vi "RoomsFGV.vi"(7 "Actions":T1, 8 "error in (no error)":errorcluster, 9 "Data In":string, 10 "Room":i32) -> (0 "error out":errorcluster, 1 "Data Out":string)   [LabVIEW 2015]
uses:
  TypeDef/RoomsActionEnum.ctl
  TypeDef/RoomsStateCluster.ctl
  LVClasses/Room/Room.lvclass
  LVClasses/Room/Room.lvclass/Room.ctl
  LVClasses/Flags/Flags.lvclass/Flags.ctl
  LVClasses/Request/SummaryJsonCluster.ctl
  LVClasses/Room/Write Bed URL.vi
  LVClasses/Room/Read Flags.lvclass.vi
  LVClasses/Room/Read RoomRequests.vi
  LVClasses/Room/Read InRoomPersonnel.vi
  LVClasses/Room/Read Beacon Id.vi
  LVClasses/Room/Read Bed URL.vi
  LVClasses/Room/Read Room Number.vi
  LVClasses/Room/Read BedVacant.vi
  LVClasses/Flags/Read State.vi
  LVClasses/Flags/Write State.vi
  LVClasses/Room/Write Flags.lvclass.vi
  LVClasses/Room/Write BedVacant.vi
  LVClasses/Room/Write RoomRequests.vi
  LVClasses/Room/Write InRoomPersonnel.vi
  <vilib>/Utility/error.llb/Error Cluster From Error Code.vi
  <vilib>/ErrorRing/Error Ring.xnode
  LVClasses/Flags/Flags.lvclass
  LVClasses/Request/Request.lvclass
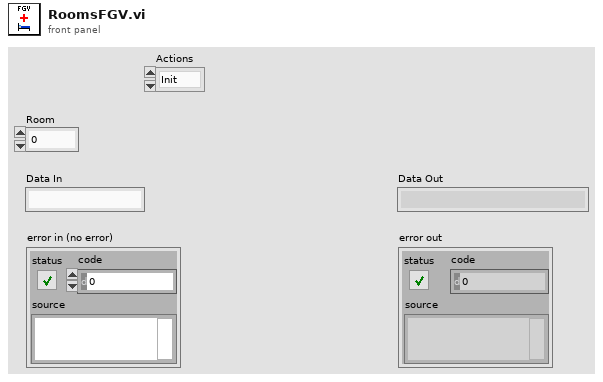
[diagram p1: front panel]
types:
  T1 = typedef "RoomsActionEnum.ctl" = enum16{"Init", "Add Room", "Remove Room", "Read Room", "Read Flag", "Read Flag State", "Write Flag State", "Read Flag Color", "Write Flag Color", "Read Bed Vacant", "Write Bed Vacant", "Read Personnel", "Add Personnel", "Remove Personnel", "Read Requests", "Add Request", "Remove Request", "Read Beacon ID", "Write Beacon ID", "Write Bed URL", "Read Bed URL", "Read Rooms Numbers", "Write Flag"}
  T2 = typedef "RoomsStateCluster.ctl" = cluster{"Rooms":refnum<class "Room.lvclass">[]}
  T3 = typedef "Request.lvclass/SummaryJsonCluster.ctl" = cluster{"RequestID":string, "EnlapsedTime":i32, "Description":string, "Alarm":bool}
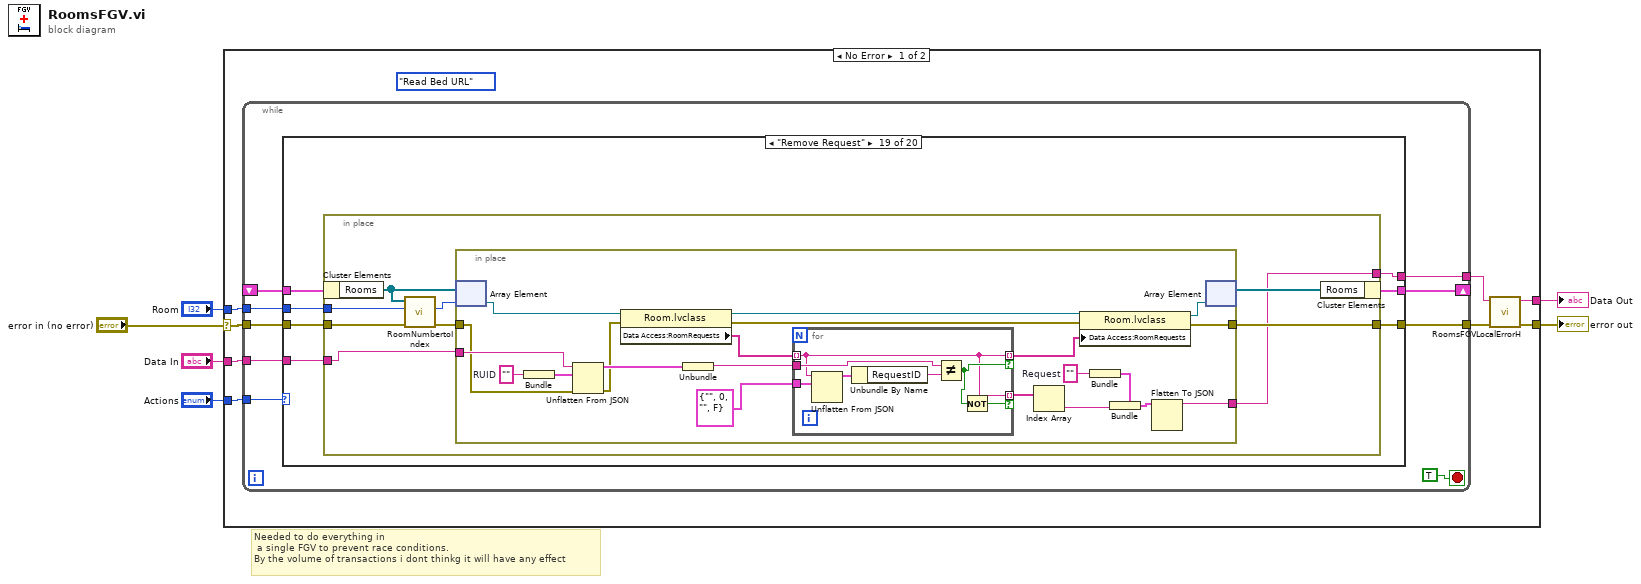
[diagram p0: block diagram]
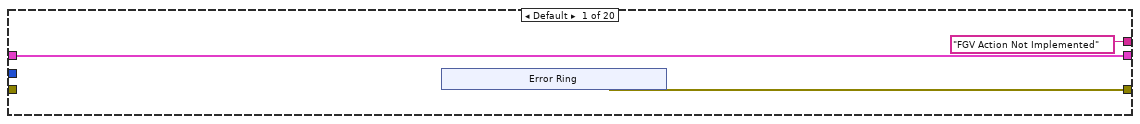
[diagram p2: hidden frame]
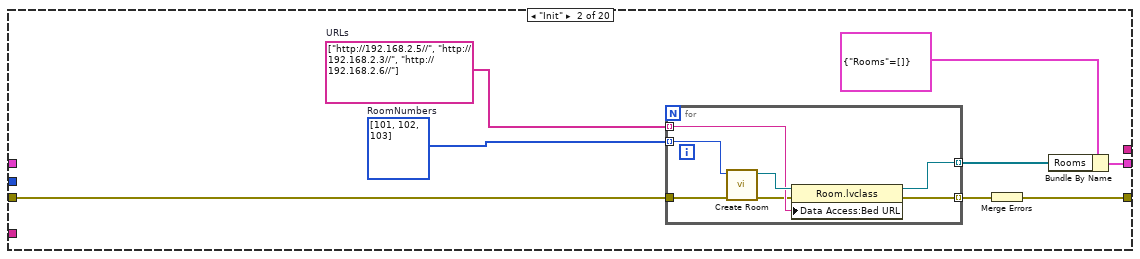
[diagram p3: hidden frame]
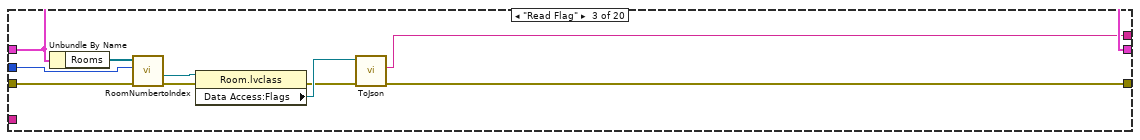
[diagram p4: hidden frame]
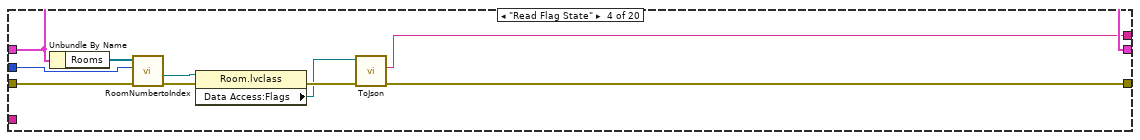
[diagram p5: hidden frame]
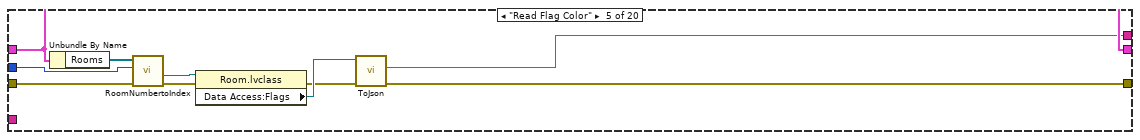
[diagram p6: hidden frame]
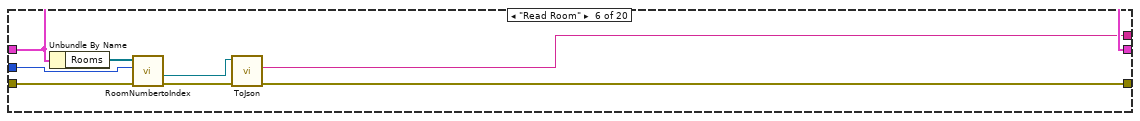
[diagram p7: hidden frame]
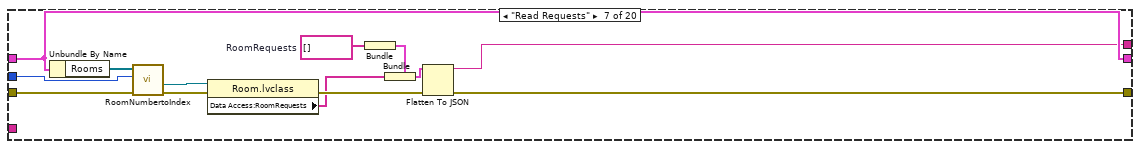
[diagram p8: hidden frame]
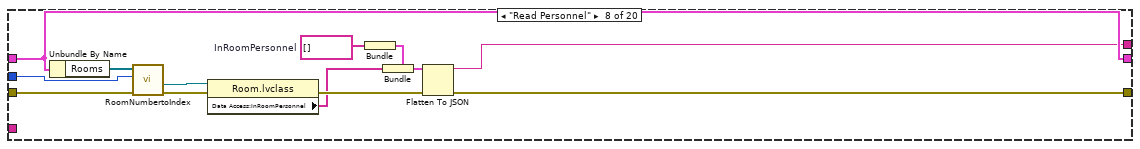
[diagram p9: hidden frame]
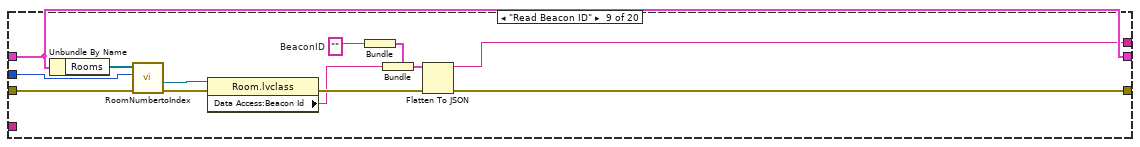
[diagram p10: hidden frame]
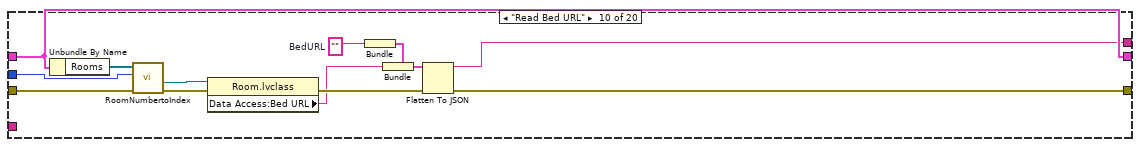
[diagram p11: hidden frame]
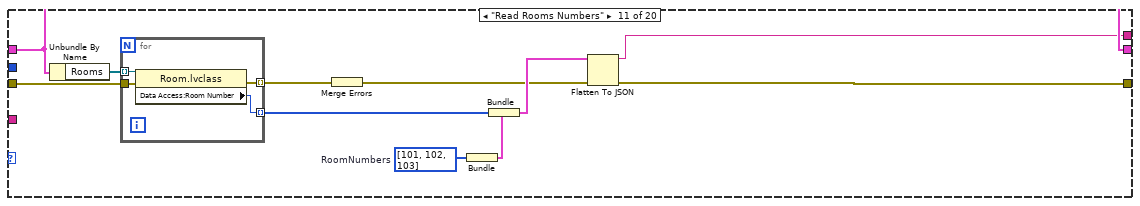
[diagram p12: hidden frame]
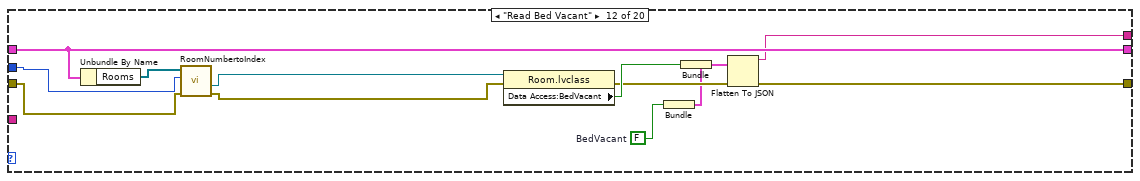
[diagram p13: hidden frame]
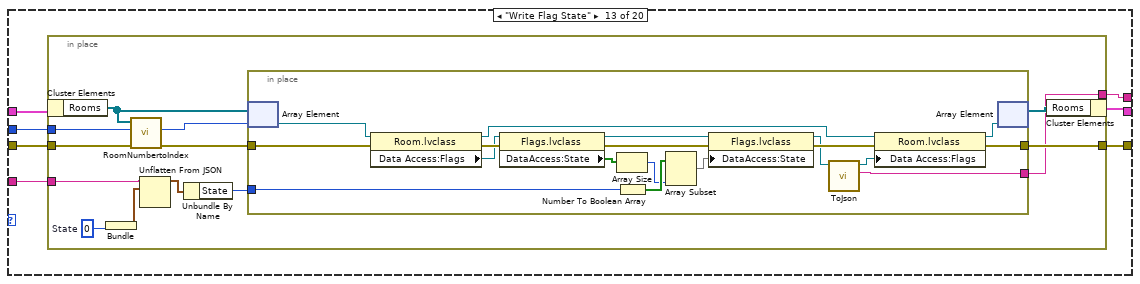
[diagram p14: hidden frame]
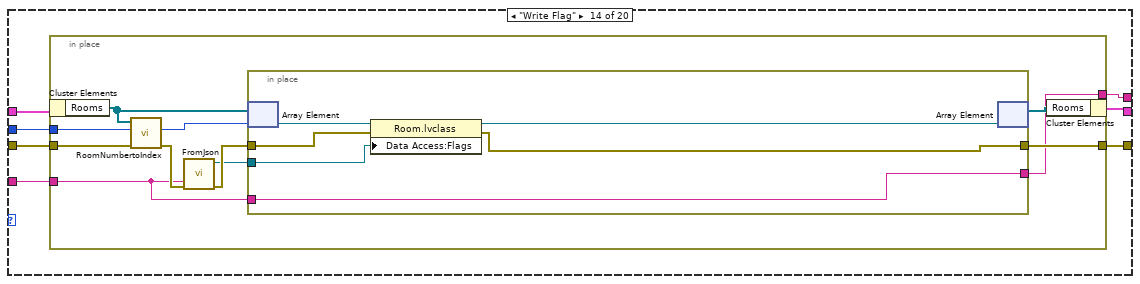
[diagram p15: hidden frame]
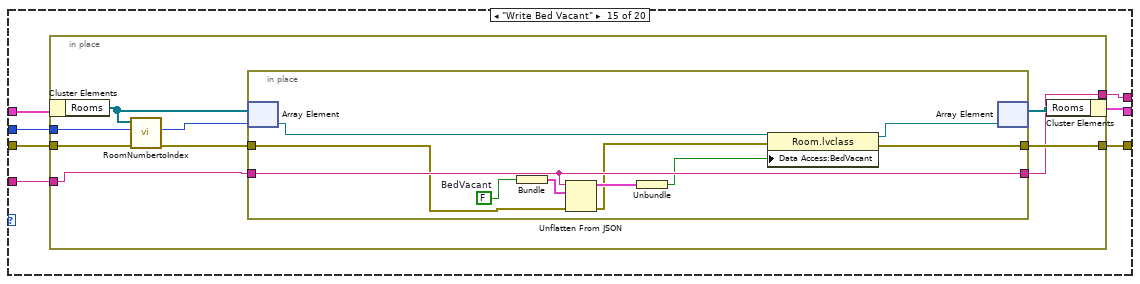
[diagram p16: hidden frame]
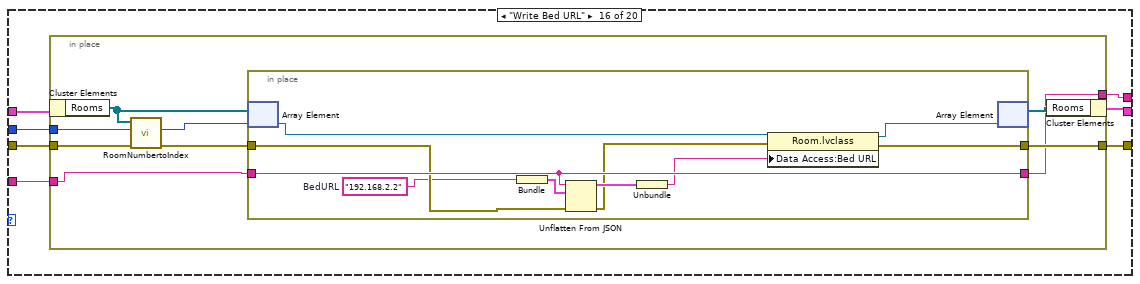
[diagram p17: hidden frame]
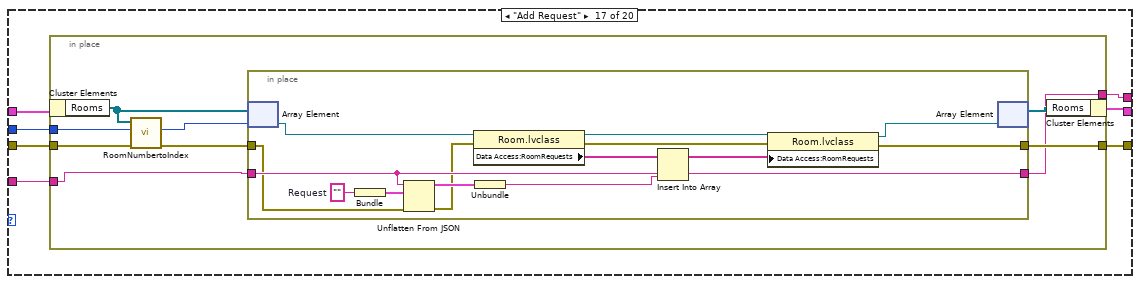
[diagram p18: hidden frame]
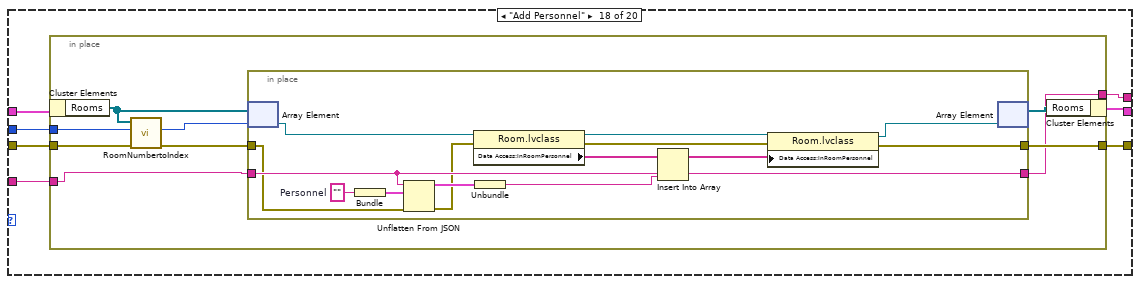
[diagram p19: hidden frame]
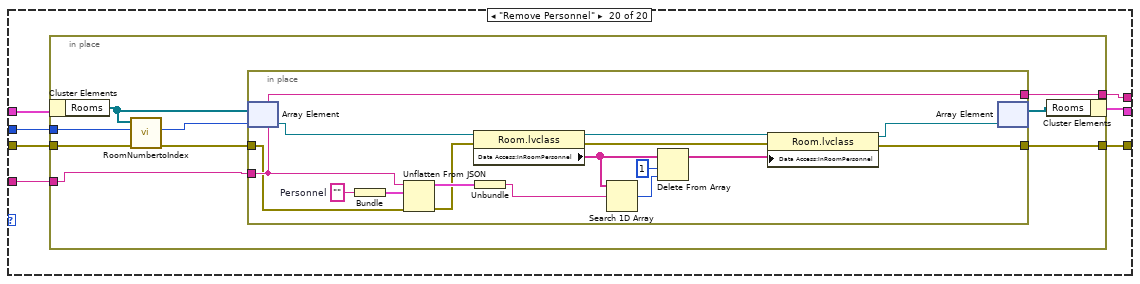
[diagram p20: hidden frame]
diagram:
  # "Needed to do everything in\n a single FGV to prevent race conditions. \nBy the volume of transactions i dont thinkg it will have any effect"
  n1 = case shown="No Error" "error in (no error)" {
    selector: "error in (no error)" -> [w11 w415]
    tunnel: "Actions" -> [w14 _]
    tunnel: "Room" -> [w13 _]
    tunnel: [w9 _] -> w4
    tunnel: "Data In" -> [w12 _]
    tunnel: [w10 w415] -> w1
    frame No Error {
      (unwired) RoomsActionEnum."Read Bed URL" ("Actions")
      n2 = while {
        shift-right: [w21] -> _
        shift-left: _ -> [w20]
        tunnel: w14 -> [w22]
        tunnel: w13 -> [w19]
        tunnel: [w18] -> w8
        tunnel: w12 -> [w17]
        tunnel: [w16] -> w7
        tunnel: w11 -> [w15]
        stop <- TRUE ("stop") stop-if-true
        n3 = case shown="\"Remove Request\"" w22 {
          tunnel: [w26 w39 w56 w66 w76 w84 w97 w110 w123 w136 w147 w164 w170 w208 w232 w258 w284 w314 w344 w388] -> w21
          tunnel: w20 -> [w26 _ w56 w66 w76 w84 w97 w110 w123 w136 w147 w164 w171 w209 w233 w259 w285 w315 w345 w389]
          tunnel: w19 -> [_ _ w55 w65 w75 w83 w96 w109 w122 w135 _ w155 w169 w207 w231 w257 w283 w313 w343 w387]
          tunnel: ["FGV Action Not Implemented" ("Data In") _ w51 w61 w71 w78 w91 w104 w117 w130 w145 w162 w168 w206 w230 w256 w282 w312 w342 w386] -> w18
          tunnel: w17 -> [_ _ _ _ _ _ _ _ _ _ _ _ w166 w204 w228 w254 w280 w310 w340 w384]
          tunnel: [w24 w32 w47 w57 w67 w77 w85 w98 w112 w125 w137 w157 w165 w203 w227 w253 w279 w309 w339 w383] -> w16
          tunnel: w15 -> [_ w33 w52 w62 w72 w81 w94 w107 w120 w133 w140 w154 w167 w205 w229 w255 w281 w311 w341 w385]
          frame Default {
            n4 = xnode "Error Ring"() -> ("error out"=w24:errorcluster)
          }
          frame "Init" {
            w36 = i32[] [101, 102, 103]  # RoomNumbers
            w35 = string[] ["http://192.168.2.5//", "http://192.168.2.3//", "http://192.168.2.6//"]  # URLs
            n5 = for {
              tunnel: w36 -> [w40] mode=indexing
              tunnel: [w45] -> w37 mode=indexing
              tunnel: w35 -> [w44] mode=indexing
              tunnel: w33 -> [w42]
              tunnel: [w41] -> w34 mode=indexing
              n6 = call "Create Room.vi"("error in"=w42, "Room Number"=w40) -> ("error out"=w43:errorcluster, "Room Ref"=w46:refnum<class "Room.lvclass">)  [unwired: 8 in]
              n7 = property class="Room.lvclass"(reference=w46, error in=w43, "Data Access:Bed URL"=w44) -> (reference out=w45:refnum<class "Room.lvclass">, error out=w41:errorcluster)
            }
            n8 = Merge Errors(w34) -> (w32:errorcluster)
            n9 = Bundle By Name(cluster=T2 {"Rooms"=[]}, "Rooms"=w37) -> (w39:T2)
          }
          frame "Read Flag" {
            n10 = Unbundle By Name(w56) -> ("Rooms"=w54:refnum<class "Room.lvclass">[])
            n11 = call "RoomNumbertoIndex.vi"("error in (no error)"=w52, "y"=w55, "Rooms In"=w54) -> ("error out"=w48:errorcluster, "Room"=w53:refnum<class "Room.lvclass">)  [unwired: 5 in, 2 out]
            n12 = property class="Room.lvclass"(reference=w53, error in=w48) -> (error out=w49:errorcluster, "Data Access:Flags"=w50:refnum<class "Flags.lvclass">)  [unwired: 1 out]
            n13 = call "ToJson.vi"("error in (no error)"=w49, "Flags in"=w50) -> ("error out"=w47:errorcluster, "String"=w51:string)  [unwired: 7 in, 1 out]
          }
          frame "Read Flag State" {
            n14 = Unbundle By Name(w66) -> ("Rooms"=w64:refnum<class "Room.lvclass">[])
            n15 = call "RoomNumbertoIndex.vi"("error in (no error)"=w62, "y"=w65, "Rooms In"=w64) -> ("error out"=w59:errorcluster, "Room"=w63:refnum<class "Room.lvclass">)  [unwired: 5 in, 2 out]
            n16 = property class="Room.lvclass"(reference=w63, error in=w59) -> (error out=w60:errorcluster, "Data Access:Flags"=w58:refnum<class "Flags.lvclass">)  [unwired: 1 out]
            n17 = call "ToJson.vi"("error in (no error)"=w60, "Flags in"=w58) -> ("error out"=w57:errorcluster, "String"=w61:string)  [unwired: 7 in, 1 out]
          }
          frame "Read Flag Color" {
            n18 = Unbundle By Name(w76) -> ("Rooms"=w74:refnum<class "Room.lvclass">[])
            n19 = call "RoomNumbertoIndex.vi"("error in (no error)"=w72, "y"=w75, "Rooms In"=w74) -> ("error out"=w68:errorcluster, "Room"=w73:refnum<class "Room.lvclass">)  [unwired: 5 in, 2 out]
            n20 = property class="Room.lvclass"(reference=w73, error in=w68) -> (error out=w69:errorcluster, "Data Access:Flags"=w70:refnum<class "Flags.lvclass">)  [unwired: 1 out]
            n21 = call "ToJson.vi"("error in (no error)"=w69, "Flags in"=w70) -> ("error out"=w67:errorcluster, "String"=w71:string)  [unwired: 7 in, 1 out]
          }
          frame "Read Room" {
            n22 = Unbundle By Name(w84) -> ("Rooms"=w82:refnum<class "Room.lvclass">[])
            n23 = call "RoomNumbertoIndex.vi"("error in (no error)"=w81, "y"=w83, "Rooms In"=w82) -> ("error out"=w80:errorcluster, "Room"=w79:refnum<class "Room.lvclass">)  [unwired: 5 in, 2 out]
            n24 = call "ToJson.vi"("error in (no error)"=w80, "Room in"=w79) -> ("error out"=w77:errorcluster, "String"=w78:string)  [unwired: 7 in, 1 out]
          }
          frame "Read Requests" {
            w88 = string[] []  # RoomRequests
            n25 = Unbundle By Name(w97) -> ("Rooms"=w95:refnum<class "Room.lvclass">[])
            n26 = call "RoomNumbertoIndex.vi"("error in (no error)"=w94, "y"=w96, "Rooms In"=w95) -> ("error out"=w92:errorcluster, "Room"=w93:refnum<class "Room.lvclass">)  [unwired: 5 in, 2 out]
            n27 = property class="Room.lvclass"(reference=w93, error in=w92) -> (error out=w90:errorcluster, "Data Access:RoomRequests"=w86:string[])  [unwired: 1 out]
            n28 = Bundle("RoomRequests"=w88) -> (w89:cluster{"RoomRequests":string[]})  [unwired: 1 in]
            n29 = Bundle(cluster=w89, "RoomRequests"=w86) -> (w87:cluster{"RoomRequests":string[]})
            n30 = Flatten To JSON(anything=w87, error in (no error)=w90) -> (JSON string=w91:string, 11:w85:errorcluster)  [unwired: 1 in]
          }
          frame "Read Personnel" {
            w101 = string[] []  # InRoomPersonnel
            n31 = Unbundle By Name(w110) -> ("Rooms"=w108:refnum<class "Room.lvclass">[])
            n32 = call "RoomNumbertoIndex.vi"("error in (no error)"=w107, "y"=w109, "Rooms In"=w108) -> ("error out"=w105:errorcluster, "Room"=w106:refnum<class "Room.lvclass">)  [unwired: 5 in, 2 out]
            n33 = property class="Room.lvclass"(reference=w106, error in=w105) -> (error out=w103:errorcluster, "Data Access:InRoomPersonnel"=w99:string[])  [unwired: 1 out]
            n34 = Bundle("InRoomPersonnel"=w101) -> (w102:cluster{"InRoomPersonnel":string[]})  [unwired: 1 in]
            n35 = Bundle(cluster=w102, "InRoomPersonnel"=w99) -> (w100:cluster{"InRoomPersonnel":string[]})
            n36 = Flatten To JSON(anything=w100, error in (no error)=w103) -> (JSON string=w104:string, 11:w98:errorcluster)  [unwired: 1 in]
          }
          frame "Read Beacon ID" {
            w111 = ""  # BeaconID
            n37 = Unbundle By Name(w123) -> ("Rooms"=w121:refnum<class "Room.lvclass">[])
            n38 = call "RoomNumbertoIndex.vi"("error in (no error)"=w120, "y"=w122, "Rooms In"=w121) -> ("error out"=w118:errorcluster, "Room"=w119:refnum<class "Room.lvclass">)  [unwired: 5 in, 2 out]
            n39 = property class="Room.lvclass"(reference=w119, error in=w118) -> (error out=w116:errorcluster, "Data Access:Beacon Id"=w113:string)  [unwired: 1 out]
            n40 = Bundle("BeaconID"=w111) -> (w115:cluster{"BeaconID":string})  [unwired: 1 in]
            n41 = Bundle(cluster=w115, "BeaconID"=w113) -> (w114:cluster{"BeaconID":string})
            n42 = Flatten To JSON(anything=w114, error in (no error)=w116) -> (JSON string=w117:string, 11:w112:errorcluster)  [unwired: 1 in]
          }
          frame "Read Bed URL" {
            w124 = ""  # BedURL
            n43 = Unbundle By Name(w136) -> ("Rooms"=w134:refnum<class "Room.lvclass">[])
            n44 = call "RoomNumbertoIndex.vi"("error in (no error)"=w133, "y"=w135, "Rooms In"=w134) -> ("error out"=w131:errorcluster, "Room"=w132:refnum<class "Room.lvclass">)  [unwired: 5 in, 2 out]
            n45 = property class="Room.lvclass"(reference=w132, error in=w131) -> (error out=w129:errorcluster, "Data Access:Bed URL"=w126:string)  [unwired: 1 out]
            n46 = Bundle("BedURL"=w124) -> (w128:cluster{"BedURL":string})  [unwired: 1 in]
            n47 = Bundle(cluster=w128, "BedURL"=w126) -> (w127:cluster{"BedURL":string})
            n48 = Flatten To JSON(anything=w127, error in (no error)=w129) -> (JSON string=w130:string, 11:w125:errorcluster)  [unwired: 1 in]
          }
          frame "Read Rooms Numbers" {
            w146 = i32[] [101, 102, 103]  # RoomNumbers
            n49 = Unbundle By Name(w147) -> ("Rooms"=w142:refnum<class "Room.lvclass">[])
            n50 = for {
              tunnel: w142 -> [w151] mode=indexing
              tunnel: [w150] -> w141 mode=indexing
              tunnel: w140 -> [w149]
              tunnel: [w148] -> w139 mode=indexing
              n51 = property class="Room.lvclass"(reference=w151, error in=w149) -> (error out=w148:errorcluster, "Data Access:Room Number"=w150:i32)  [unwired: 1 out]
            }
            n52 = Merge Errors(w139) -> (w138:errorcluster)
            n53 = Bundle("RoomNumbers"=w146) -> (w144:cluster{"RoomNumbers":i32[]})  [unwired: 1 in]
            n54 = Bundle(cluster=w144, "RoomNumbers"=w141) -> (w143:cluster{"RoomNumbers":i32[]})
            n55 = Flatten To JSON(anything=w143, error in (no error)=w138) -> (JSON string=w145:string, 11:w137:errorcluster)  [unwired: 1 in]
          }
          frame "Read Bed Vacant" {
            w159 = FALSE  # BedVacant
            n56 = Unbundle By Name(w164) -> ("Rooms"=w156:refnum<class "Room.lvclass">[])
            n57 = call "RoomNumbertoIndex.vi"("error in (no error)"=w154, "y"=w155, "Rooms In"=w156) -> ("error out"=w153:errorcluster, "Room"=w152:refnum<class "Room.lvclass">)  [unwired: 5 in, 2 out]
            n58 = property class="Room.lvclass"(reference=w152, error in=w153) -> (error out=w160:errorcluster, "Data Access:BedVacant"=w161:bool)  [unwired: 1 out]
            n59 = Bundle("BedVacant"=w159) -> (w158:cluster{"BedVacant":bool})  [unwired: 1 in]
            n60 = Bundle(cluster=w158, "BedVacant"=w161) -> (w163:cluster{"BedVacant":bool})
            n61 = Flatten To JSON(anything=w163, error in (no error)=w160) -> (JSON string=w162:string, 11:w157:errorcluster)  [unwired: 1 in]
          }
          frame "Write Flag State" {
            n62 = in-place {
              in-place-border: w169 -> [w182]
              in-place-border: [w178] -> w168
              in-place-border: w167 -> [w180]
              in-place-border: [w179] -> w165
              in-place-border: w166 -> [w176]
              w175 = 0  # State
              n63 = in-place-cluster #1(w171) -> ("Rooms"=w183:refnum<class "Room.lvclass">[])
              n64 = Bundle("State"=w175) -> (w174:cluster{"State":i32})  [unwired: 1 in]
              n65 = call "RoomNumbertoIndex.vi"("error in (no error)"=w180, "y"=w182, "Rooms In"=w183) -> ("error out"=w177:errorcluster, "Index"=w181:i32)  [unwired: 5 in, 2 out]
              n66 = Unflatten From JSON(JSON string=w176, type and defaults=w174) -> (value=w173:cluster{"State":i32})  [unwired: 5 in, 1 out]
              n67 = Unbundle By Name(w173) -> ("State"=w172:i32)
              n68 = in-place {
                in-place-border: w177 -> [w197]
                in-place-border: [w189] -> w179
                in-place-border: w172 -> [w200]
                in-place-border: [w185] -> w178
                n69 = in-place-array #2(w183, w181) -> (w192:refnum<class "Room.lvclass">)
                n70 = property class="Room.lvclass"(reference=w192, error in=w197) -> (reference out=w191:refnum<class "Room.lvclass">, error out=w198:errorcluster, "Data Access:Flags"=w196:refnum<class "Flags.lvclass">)
                n71 = property class="Flags.lvclass"(reference=w196, error in=w198) -> (reference out=w188:refnum<class "Flags.lvclass">, error out=w199:errorcluster, "DataAccess:State"=w195:bool[])
                n72 = Array Size(array=w195) -> (size(s)=w194:i32)
                n73 = Number To Boolean Array(number=w200) -> (Boolean array=w201:bool[])
                n74 = Array Subset(array=w201, length=w194) -> (w193:bool[])  [unwired: 1 in]
                n75 = property class="Flags.lvclass"(reference=w188, error in=w199, "DataAccess:State"=w193) -> (reference out=w187:refnum<class "Flags.lvclass">, error out=w190:errorcluster)
                n76 = call "ToJson.vi"("Flags in"=w187) -> ("String"=w185:string, "Flags out"=w186:refnum<class "Flags.lvclass">)  [unwired: 8 in, 1 out]
                n77 = property class="Room.lvclass"(reference=w191, error in=w190, "Data Access:Flags"=w186) -> (reference out=w202:refnum<class "Room.lvclass">, error out=w189:errorcluster)
                n78 = in-place-array #2(w202) -> (w184:refnum<class "Room.lvclass">[])  [unwired: 1 out]
              }
              n79 = in-place-cluster #1("Rooms"=w184) -> (w170:T2)
            }
          }
          frame "Write Flag" {
            n80 = in-place {
              in-place-border: w207 -> [w218]
              in-place-border: [w214] -> w206
              in-place-border: w205 -> [w216]
              in-place-border: [w215] -> w203
              in-place-border: w204 -> [w211]
              n81 = in-place-cluster #3(w209) -> ("Rooms"=w219:refnum<class "Room.lvclass">[])
              n82 = call "RoomNumbertoIndex.vi"("error in (no error)"=w216, "y"=w218, "Rooms In"=w219) -> ("error out"=w213:errorcluster, "Index"=w217:i32)  [unwired: 5 in, 2 out]
              n83 = call "FromJson.vi"("error in (no error)"=w213, "String"=w211) -> ("error out"=w212:errorcluster, "Flags out"=w210:refnum<class "Flags.lvclass">)  [unwired: 8 in]
              n84 = in-place {
                in-place-border: w212 -> [w226]
                in-place-border: [w223] -> w215
                in-place-border: [w224] -> w214
                in-place-border: w211 -> [w224]
                in-place-border: w210 -> [w221]
                n85 = in-place-array #4(w219, w217) -> (w225:refnum<class "Room.lvclass">)
                n86 = property class="Room.lvclass"(reference=w225, error in=w226, "Data Access:Flags"=w221) -> (reference out=w222:refnum<class "Room.lvclass">, error out=w223:errorcluster)
                n87 = in-place-array #4(w222) -> (w220:refnum<class "Room.lvclass">[])  [unwired: 1 out]
              }
              n88 = in-place-cluster #3("Rooms"=w220) -> (w208:T2)
            }
          }
          frame "Write Bed Vacant" {
            n89 = in-place {
              in-place-border: w231 -> [w240]
              in-place-border: [w236] -> w230
              in-place-border: w229 -> [w238]
              in-place-border: [w237] -> w227
              in-place-border: w228 -> [w235]
              n90 = in-place-cluster #5(w233) -> ("Rooms"=w241:refnum<class "Room.lvclass">[])
              n91 = call "RoomNumbertoIndex.vi"("error in (no error)"=w238, "y"=w240, "Rooms In"=w241) -> ("error out"=w234:errorcluster, "Index"=w239:i32)  [unwired: 5 in, 2 out]
              n92 = in-place {
                in-place-border: w234 -> [w243]
                in-place-border: [w252] -> w237
                in-place-border: [w249] -> w236
                in-place-border: w235 -> [w249]
                w246 = FALSE  # BedVacant
                n93 = in-place-array #6(w241, w239) -> (w245:refnum<class "Room.lvclass">)
                n94 = Bundle("BedVacant"=w246) -> (w250:cluster{"BedVacant":bool})  [unwired: 1 in]
                n95 = Unflatten From JSON(JSON string=w249, type and defaults=w250, error in (no error)=w243) -> (value=w248:cluster{"BedVacant":bool}, error out=w244:errorcluster)  [unwired: 4 in]
                n96 = Unbundle(w248) -> ("BedVacant"=w247:bool)
                n97 = property class="Room.lvclass"(reference=w245, error in=w244, "Data Access:BedVacant"=w247) -> (reference out=w251:refnum<class "Room.lvclass">, error out=w252:errorcluster)
                n98 = in-place-array #6(w251) -> (w242:refnum<class "Room.lvclass">[])  [unwired: 1 out]
              }
              n99 = in-place-cluster #5("Rooms"=w242) -> (w232:T2)
            }
          }
          frame "Write Bed URL" {
            n100 = in-place {
              in-place-border: w257 -> [w266]
              in-place-border: [w262] -> w256
              in-place-border: w255 -> [w264]
              in-place-border: [w263] -> w253
              in-place-border: w254 -> [w261]
              n101 = in-place-cluster #7(w259) -> ("Rooms"=w267:refnum<class "Room.lvclass">[])
              n102 = call "RoomNumbertoIndex.vi"("error in (no error)"=w264, "y"=w266, "Rooms In"=w267) -> ("error out"=w260:errorcluster, "Index"=w265:i32)  [unwired: 5 in, 2 out]
              n103 = in-place {
                in-place-border: w260 -> [w270]
                in-place-border: [w278] -> w263
                in-place-border: [w275] -> w262
                in-place-border: w261 -> [w275]
                w269 = "192.168.2.2"  # BedURL
                n104 = in-place-array #8(w267, w265) -> (w272:refnum<class "Room.lvclass">)
                n105 = Bundle("BedURL"=w269) -> (w276:cluster{"BedURL":string})  [unwired: 1 in]
                n106 = Unflatten From JSON(JSON string=w275, type and defaults=w276, error in (no error)=w270) -> (value=w274:cluster{"BedURL":string}, error out=w271:errorcluster)  [unwired: 4 in]
                n107 = Unbundle(w274) -> ("BedURL"=w273:string)
                n108 = property class="Room.lvclass"(reference=w272, error in=w271, "Data Access:Bed URL"=w273) -> (reference out=w277:refnum<class "Room.lvclass">, error out=w278:errorcluster)
                n109 = in-place-array #8(w277) -> (w268:refnum<class "Room.lvclass">[])  [unwired: 1 out]
              }
              n110 = in-place-cluster #7("Rooms"=w268) -> (w258:T2)
            }
          }
          frame "Add Request" {
            n111 = in-place {
              in-place-border: w283 -> [w292]
              in-place-border: [w288] -> w282
              in-place-border: w281 -> [w290]
              in-place-border: [w289] -> w279
              in-place-border: w280 -> [w287]
              n112 = in-place-cluster #9(w285) -> ("Rooms"=w293:refnum<class "Room.lvclass">[])
              n113 = call "RoomNumbertoIndex.vi"("error in (no error)"=w290, "y"=w292, "Rooms In"=w293) -> ("error out"=w286:errorcluster, "Index"=w291:i32)  [unwired: 5 in, 2 out]
              n114 = in-place {
                in-place-border: w286 -> [w302]
                in-place-border: [w308] -> w289
                in-place-border: [w305] -> w288
                in-place-border: w287 -> [w305]
                w301 = ""  # Request
                n115 = in-place-array #10(w293, w291) -> (w303:refnum<class "Room.lvclass">)
                n116 = Bundle("Request"=w301) -> (w306:cluster{"Request":string})  [unwired: 1 in]
                n117 = Unflatten From JSON(JSON string=w305, type and defaults=w306, error in (no error)=w302) -> (value=w304:cluster{"Request":string}, error out=w299:errorcluster)  [unwired: 4 in]
                n118 = property class="Room.lvclass"(reference=w303, error in=w299) -> (reference out=w300:refnum<class "Room.lvclass">, error out=w298:errorcluster, "Data Access:RoomRequests"=w297:string[])
                n119 = Unbundle(w304) -> ("Request"=w295:string)
                n120 = Insert Into Array(array=w297, new element=w295) -> (w296:string[])  [unwired: 1 in]
                n121 = property class="Room.lvclass"(reference=w300, error in=w298, "Data Access:RoomRequests"=w296) -> (reference out=w307:refnum<class "Room.lvclass">, error out=w308:errorcluster)
                n122 = in-place-array #10(w307) -> (w294:refnum<class "Room.lvclass">[])  [unwired: 1 out]
              }
              n123 = in-place-cluster #9("Rooms"=w294) -> (w284:T2)
            }
          }
          frame "Add Personnel" {
            n124 = in-place {
              in-place-border: w313 -> [w322]
              in-place-border: [w318] -> w312
              in-place-border: w311 -> [w320]
              in-place-border: [w319] -> w309
              in-place-border: w310 -> [w317]
              n125 = in-place-cluster #11(w315) -> ("Rooms"=w323:refnum<class "Room.lvclass">[])
              n126 = call "RoomNumbertoIndex.vi"("error in (no error)"=w320, "y"=w322, "Rooms In"=w323) -> ("error out"=w316:errorcluster, "Index"=w321:i32)  [unwired: 5 in, 2 out]
              n127 = in-place {
                in-place-border: w316 -> [w332]
                in-place-border: [w338] -> w319
                in-place-border: [w335] -> w318
                in-place-border: w317 -> [w335]
                w331 = ""  # Personnel
                n128 = in-place-array #12(w323, w321) -> (w333:refnum<class "Room.lvclass">)
                n129 = Bundle("Personnel"=w331) -> (w336:cluster{"Personnel":string})  [unwired: 1 in]
                n130 = Unflatten From JSON(JSON string=w335, type and defaults=w336, error in (no error)=w332) -> (value=w334:cluster{"Personnel":string}, error out=w329:errorcluster)  [unwired: 4 in]
                n131 = property class="Room.lvclass"(reference=w333, error in=w329) -> (reference out=w330:refnum<class "Room.lvclass">, error out=w328:errorcluster, "Data Access:InRoomPersonnel"=w327:string[])
                n132 = Unbundle(w334) -> ("Personnel"=w325:string)
                n133 = Insert Into Array(array=w327, new element=w325) -> (w326:string[])  [unwired: 1 in]
                n134 = property class="Room.lvclass"(reference=w330, error in=w328, "Data Access:InRoomPersonnel"=w326) -> (reference out=w337:refnum<class "Room.lvclass">, error out=w338:errorcluster)
                n135 = in-place-array #12(w337) -> (w324:refnum<class "Room.lvclass">[])  [unwired: 1 out]
              }
              n136 = in-place-cluster #11("Rooms"=w324) -> (w314:T2)
            }
          }
          frame "Remove Request" {
            n137 = in-place {
              in-place-border: w343 -> [w352]
              in-place-border: [w346] -> w342
              in-place-border: w341 -> [w350]
              in-place-border: [w349] -> w339
              in-place-border: w340 -> [w348]
              n138 = in-place-cluster #13(w345) -> ("Rooms"=w353:refnum<class "Room.lvclass">[])
              n139 = call "RoomNumbertoIndex.vi"("error in (no error)"=w350, "y"=w352, "Rooms In"=w353) -> ("error out"=w347:errorcluster, "Index"=w351:i32)  [unwired: 5 in, 2 out]
              n140 = in-place {
                in-place-border: w347 -> [w369]
                in-place-border: [w375] -> w349
                in-place-border: w348 -> [w372]
                in-place-border: [w355] -> w346
                w360 = ""  # Request
                w368 = ""  # RUID
                n141 = in-place-array #14(w353, w351) -> (w370:refnum<class "Room.lvclass">)
                n142 = Bundle("RUID"=w368) -> (w373:cluster{"RUID":string})  [unwired: 1 in]
                n143 = Unflatten From JSON(JSON string=w372, type and defaults=w373, error in (no error)=w369) -> (value=w371:cluster{"RUID":string}, error out=w366:errorcluster)  [unwired: 4 in]
                n144 = property class="Room.lvclass"(reference=w370, error in=w366) -> (reference out=w367:refnum<class "Room.lvclass">, error out=w365:errorcluster, "Data Access:RoomRequests"=w363:string[])
                n145 = Unbundle(w371) -> ("RUID"=w361:string)
                n146 = for {
                  tunnel: [w376] -> w364 mode=indexing if=w377
                  tunnel: w363 -> [w376] mode=indexing
                  tunnel: T3 {"RequestID"="", "EnlapsedTime"=0, "Description"="", "Alarm"=FALSE} ("RequestTable") -> [w382]
                  tunnel: w361 -> [w379]
                  tunnel: [w376] -> w357 mode=indexing if=w378
                  n147 = Unflatten From JSON(JSON string=w376, type and defaults=w382) -> (value=w381:T3)  [unwired: 5 in, 1 out]
                  n148 = Unbundle By Name(w381) -> ("RequestID"=w380:string)
                  n149 = Not Equal?(x=w379, y=w380) -> (x != y?=w377:bool)
                  n150 = Not(x=w377) -> (.not. x?=w378:bool)
                }
                n151 = Index Array(array=w357) -> (element=w359:string)  [unwired: 1 in]
                n152 = property class="Room.lvclass"(reference=w367, error in=w365, "Data Access:RoomRequests"=w364) -> (reference out=w374:refnum<class "Room.lvclass">, error out=w375:errorcluster)
                n153 = Bundle("Request"=w360) -> (w356:cluster{"Request":string})  [unwired: 1 in]
                n154 = Bundle(cluster=w356, "Request"=w359) -> (w358:cluster{"Request":string})
                n155 = Flatten To JSON(anything=w358) -> (JSON string=w355:string)  [unwired: 2 in, 1 out]
                n156 = in-place-array #14(w374) -> (w354:refnum<class "Room.lvclass">[])  [unwired: 1 out]
              }
              n157 = in-place-cluster #13("Rooms"=w354) -> (w344:T2)
            }
          }
          frame "Remove Personnel" {
            n158 = in-place {
              in-place-border: w387 -> [w396]
              in-place-border: [w392] -> w386
              in-place-border: w385 -> [w394]
              in-place-border: [w393] -> w383
              in-place-border: w384 -> [w391]
              n159 = in-place-cluster #15(w389) -> ("Rooms"=w397:refnum<class "Room.lvclass">[])
              n160 = call "RoomNumbertoIndex.vi"("error in (no error)"=w394, "y"=w396, "Rooms In"=w397) -> ("error out"=w390:errorcluster, "Index"=w395:i32)  [unwired: 5 in, 2 out]
              n161 = in-place {
                in-place-border: w390 -> [w408]
                in-place-border: [w414] -> w393
                in-place-border: [w411] -> w392
                in-place-border: w391 -> [w411]
                w407 = ""  # Personnel
                n162 = in-place-array #16(w397, w395) -> (w409:refnum<class "Room.lvclass">)
                n163 = Bundle("Personnel"=w407) -> (w412:cluster{"Personnel":string})  [unwired: 1 in]
                n164 = Unflatten From JSON(JSON string=w411, type and defaults=w412, error in (no error)=w408) -> (value=w410:cluster{"Personnel":string}, error out=w405:errorcluster)  [unwired: 4 in]
                n165 = property class="Room.lvclass"(reference=w409, error in=w405) -> (reference out=w406:refnum<class "Room.lvclass">, error out=w404:errorcluster, "Data Access:InRoomPersonnel"=w401:string[])
                n166 = Unbundle(w410) -> ("Personnel"=w402:string)
                n167 = Search 1D Array(1D array=w401, element=w402) -> (index of element=w400:i32)  [unwired: 1 in]
                n168 = Delete From Array(array=w401, length=1, index=w400) -> (array with subset deleted=w403:string[])  [unwired: 1 out]
                n169 = property class="Room.lvclass"(reference=w406, error in=w404, "Data Access:InRoomPersonnel"=w403) -> (reference out=w413:refnum<class "Room.lvclass">, error out=w414:errorcluster)
                n170 = in-place-array #16(w413) -> (w398:refnum<class "Room.lvclass">[])  [unwired: 1 out]
              }
              n171 = in-place-cluster #15("Rooms"=w398) -> (w388:T2)
            }
          }
        }
      }
      n172 = call "RoomsFGVLocalErrorH.vi"("error in (no error)"=w7, "String in"=w8) -> ("error out"=w10:errorcluster, "String out"=w9:string)  [unwired: 8 in]
    }
    frame Error {
    }
  }
  "Data Out" <- w4
  "error out" <- w1
